vi "p5posicion arduino.vi"() -> ()   [LabVIEW 2017]
uses:
  <vilib>/LabVIEW Interface for Arduino/Type Defs/Connection Type.ctl
  <vilib>/LabVIEW Interface for Arduino/Type Defs/Board Type.ctl
  <vilib>/LabVIEW Interface for Arduino/LabVIEW Interface for Arduino.lvlib
panel:
  in  "stop":bool
  out "Numeric":i32
  out "Angle (Degrees)":u8=15
  in  "Dial":dbl(knob) scale=0.0..180.0
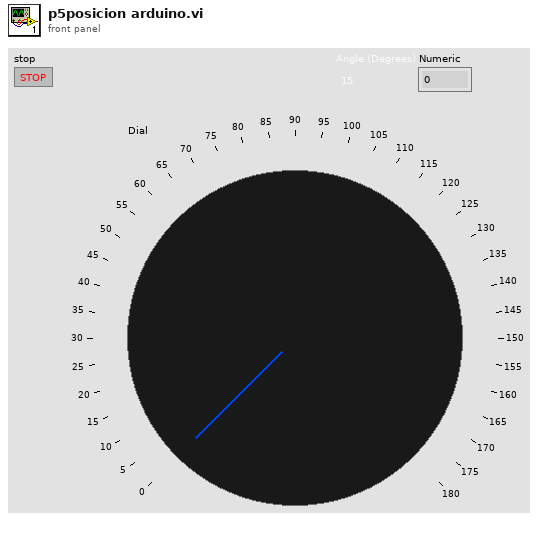
[diagram p1: front panel]
types:
  T1 = typedef "LabVIEW Interface for Arduino.lvlib/Board Type.ctl" = enum16{"Uno", "Dimuelanove w/Atmega 328", "Mega 2560"}
  T2 = typedef "LabVIEW Interface for Arduino.lvlib/Connection Type.ctl" = enum8{"USB / Serial", "XBEE", "BlueSmirf (Bluetooth)"}
  T3 = typedef "LabVIEW Interface for Arduino.lvlib/Arduino Resource.ctl" = cluster{"VISA resource":refnum<visa-resource-name>, "Board Type":T1, "Connection Type":enum8{"USB / Serial"}, "Bytes Per Packet (15)":u8}
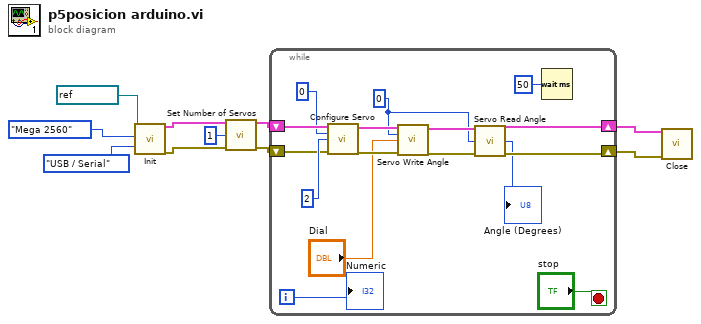
[diagram p0: block diagram]
diagram:
  n1 = call <vilib>:"Init.vi"("VISA resource"=refnum<visa-resource-name> "COM3", "Board Type (Uno)"=Board_Type."Mega 2560", "Connection Type (USB/Serial)"=Connection_Type."USB / Serial") -> ("Arduino Resource"=w5:T3, "error out"=w4:errorcluster)  [unwired: 15 in]
  n2 = call <vilib>:"Set Number of Servos.vi"("Arduino Resource"=w5, "Number Of Servos (1)"=u8 1, "error in"=w4) -> ("Arduino Resource"=w10:T3, "error out"=w9:errorcluster)  [unwired: 11 in]
  n3 = while {
    shift-right: [w16] -> w7
    shift-left: w10 -> [w26]
    shift-right: [w17] -> w8
    shift-left: w9 -> [w23]
    i -> [w13]
    stop <- "stop" stop-if-true
    w19 = u8 0 ("Servo Number")
    n4 = call <vilib>:"Configure Servo.vi"("Arduino Resource"=w26, "Servo Number (0)"=u8 0, "DIO Pin (2)"=u8 2, "error in"=w23) -> ("Arduino Resource"=w22:T3, "error out"=w21:errorcluster)  [unwired: 10 in]
    n5 = call <vilib>:"Servo Write Angle.vi"("Arduino Resource"=w22, "Servo Number"=w19, "Angle (Degrees)"="Dial", "error in"=w21) -> ("Arduino Resource"=w20:T3, "error out"=w18:errorcluster)  [unwired: 10 in]
    n6 = call <vilib>:"Servo Read Angle.vi"("Arduino Resource"=w20, "Servo Number"=w19, "error in"=w18) -> ("Arduino Resource"=w16:T3, "Angle (Degrees)"=→"Angle (Degrees)":u8, "error out"=w17:errorcluster)  [unwired: 10 in]
    n7 = Wait (ms)(milliseconds to wait=u32 50) -> ()  [unwired: 1 out]
    "Numeric" <- w13
  }
  n8 = call <vilib>:"Close.vi"("Arduino Resource"=w7, "error in"=w8) -> ()  [unwired: 13 in, 1 out]
